vi "Write VISA.vi"(8 "error in (no error)":errorcluster, 10 "VISA":string, 11 "T560Session in":refnum<class "T560Session.lvclass">) -> (0 "error out":errorcluster, 3 "T560Session out":refnum<class "T560Session.lvclass">)   [LabVIEW 2020, in "T560Session.lvclass"]
uses:
  T560Session.lvclass
  T560Session.lvclass/T560Session.ctl
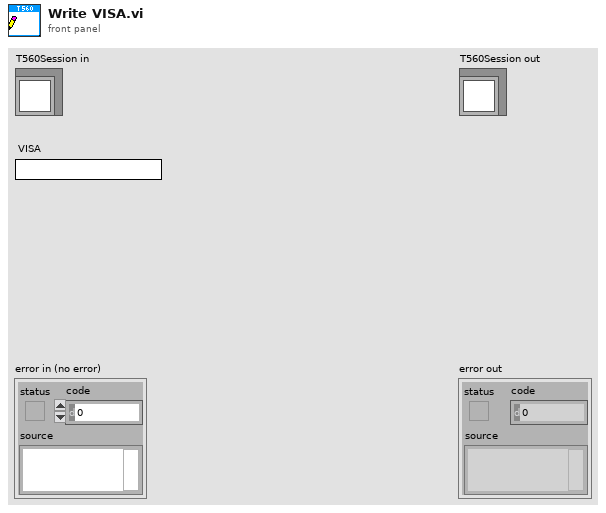
[diagram p1: front panel]
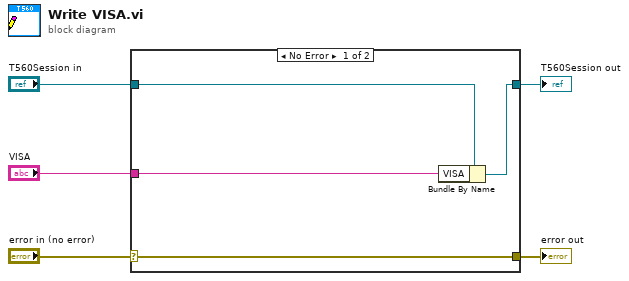
[diagram p0: block diagram]
diagram:
  n1 = case shown="No Error" "error in (no error)" {
    selector: "error in (no error)" -> [w9 w10]
    tunnel: [w9 w10] -> w4
    tunnel: [w7 w11] -> w2
    tunnel: "T560Session in" -> [w8 w11]
    tunnel: "VISA" -> [w6 _]
    frame No Error {
      n2 = Bundle By Name(cluster=w8, "VISA"=w6) -> (w7:refnum<class "T560Session.lvclass">)
    }
    frame Error {
    }
  }
  "error out" <- w4
  "T560Session out" <- w2
